vi "clearpath_set_differential_speeds.vi"(0 "ClearpathComm":T1, 1 "Right Accel":dbl=0.5, 2 "Left Accel":dbl=0.5, 3 "Right Speed":dbl, 4 "Left Speed":dbl) -> ()   [LabVIEW 2010, in "clearpath_interface.lvlib"]
doc: "Formats a Set Differential Speeds command (0x200) to set desired left and right side wheel speeds, given speeds in m/s and accelerations in m/s^2. An acceleration of 0.5 m/s^2 or slower is recommended. Uses the onboard Clearpath library to perform the actual message formatting."
uses:
  clearpath_interface.lvlib
  cwrap_cRIO.dll
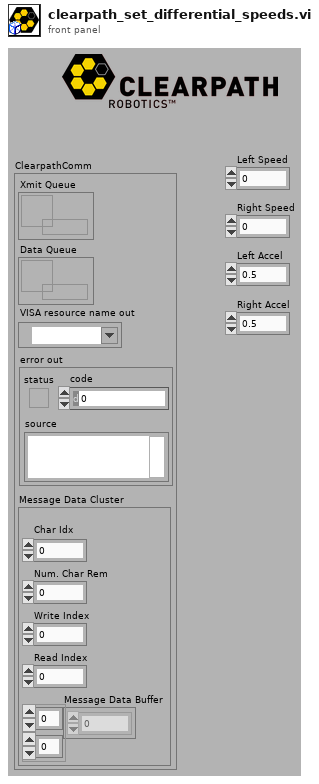
[diagram p1: front panel]
types:
  T1 = cluster{"Xmit Queue":refnum<queue>, "Data Queue":refnum<queue>, "VISA resource name out":refnum<visa-resource-name>, "error out":errorcluster, "Message Data Cluster":cluster{"\nChar Idx":u8, "Num. Char Rem":u8, "Write Index":u8, "Read Index":u8, "Message Data Buffer":u8[][]}}
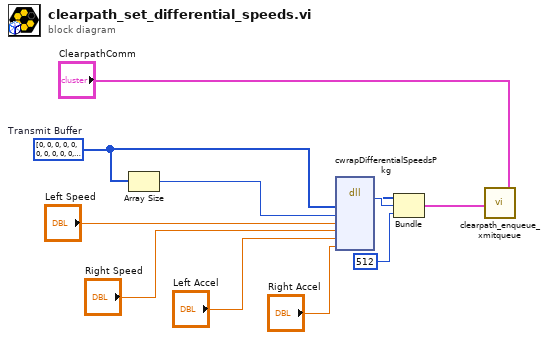
[diagram p0: block diagram]
diagram:
  w8 = u8[] [0, 0, 0, 0, 0, 0, 0, 0, 0, 0, 0, 0, 0, 0, 0, 0, 0, 0, 0, 0, 0, 0, 0, 0, 0, 0, 0, 0, 0, 0, 1, 0, 0, 0, 5]  # Transmit Buffer
  n1 = Array Size(array=w8) -> (size(s)=w9:i32)
  n2 = dll-call lib="cwrap_cRIO.*" fn="cwrapDifferentialSpeedsPkg"("buf"=w8, "buf_size"=w9, "l_speed"="Left Speed", "r_speed"="Right Speed", "l_accel"="Left Accel", "r_accel"="Right Accel") -> ("return type"=w11:i32, "buf"=w10:u8[])  [unwired: 8 in, 2 out]
  n3 = Bundle("buf"=w10, "return type"=w11, 512) -> (w2:cluster{"buf":u8[], "return type":i32, i32})  [unwired: 1 in]
  n4 = call "clearpath_enqueue_xmitqueue.vi"("ClearpathComm"="ClearpathComm", "Cluster"=w2) -> ()
